vi "Modbus RT Driver VI Modbus - Read Write Items.vi"(5 "DEBUG RT-FIFOs Indexes":T1[](array[typedef]), 7 "DEBUG Modbus Items":T3[](array[typedef]), 8 "error in (no error)":errorcluster, 9 "Inputs In":dbl[](array[numeric]), 10 "Outputs In":dbl[](array[numeric]), 11 "ModbusPharLap.lvlibp:Modbus API":refnum<class "Modbus API.lvclass">) -> (0 "error out":errorcluster, 2 "Outputs Out":dbl[](array[numeric]), 3 "ModbusPharLap.lvlibp:Modbus API":refnum<class "Modbus API.lvclass">)   [LabVIEW 2014, in "Modbus Engine.lvlib"]
uses:
  Modbus Engine.lvlib
  XML Deserializer/XML VIs/API/Controls/Modbus_Items.ctl
  XML Deserializer/XML VIs/API/Controls/Modbus_Item_Type.ctl
  Shared/FIFO Indexes.ctl
  <vilib>/NI Veristand/Custom Device API/Custom Device Channel Type.ctl
  ModbusPharLap.lvlibp/Modbus Library/API/Modbus API.lvclass
  ModbusPharLap.lvlibp/Modbus Library/API/Slave/Modbus Slave.lvclass
  Shared/Modbus Shared.lvlib
  <vilib>/NI Veristand/Custom Device API/Custom Device API.lvlib
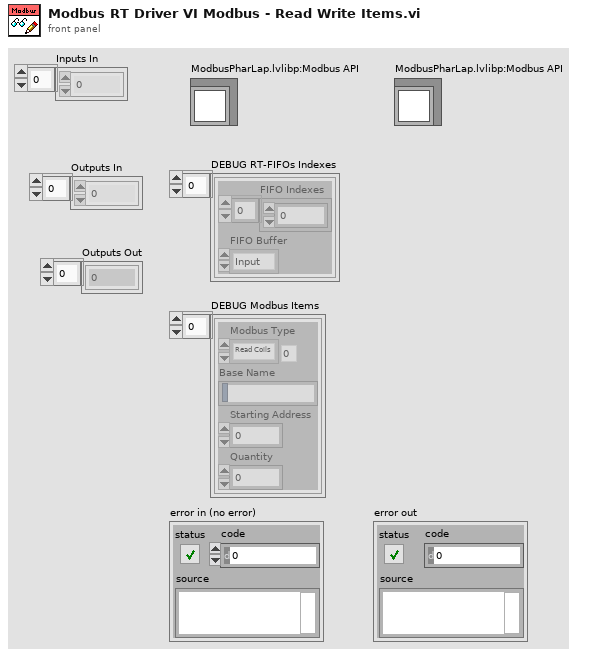
[diagram p1: front panel]
types:
  T1 = typedef "Modbus Shared.lvlib/FIFO Indexes.ctl" = cluster{"FIFO Indexes":i32[], "FIFO Buffer":T2}
  T2 = typedef "Custom Device API.lvlib/Custom Device Channel Type.ctl" = enum16{"Input", "Output"}
  T3 = typedef "Modbus Shared.lvlib/Modbus_Items.ctl" = cluster{"Modbus Type":T4, "Base Name":string, "Starting Address":u16, "Quantity":u16}
  T4 = typedef "Modbus Shared.lvlib/Modbus_Item_Type.ctl" = enum16{"Read Coils", "Read Discrete Inputs", "Read Holding Registers", "Read Input Registers", "Write Multiple Coils", "Write Multiple Holding Registers", "Write Single Coil", "Write Single Holding Register", "Write Multiple Discrete Inputs", "Write Multiple Input Registers"}
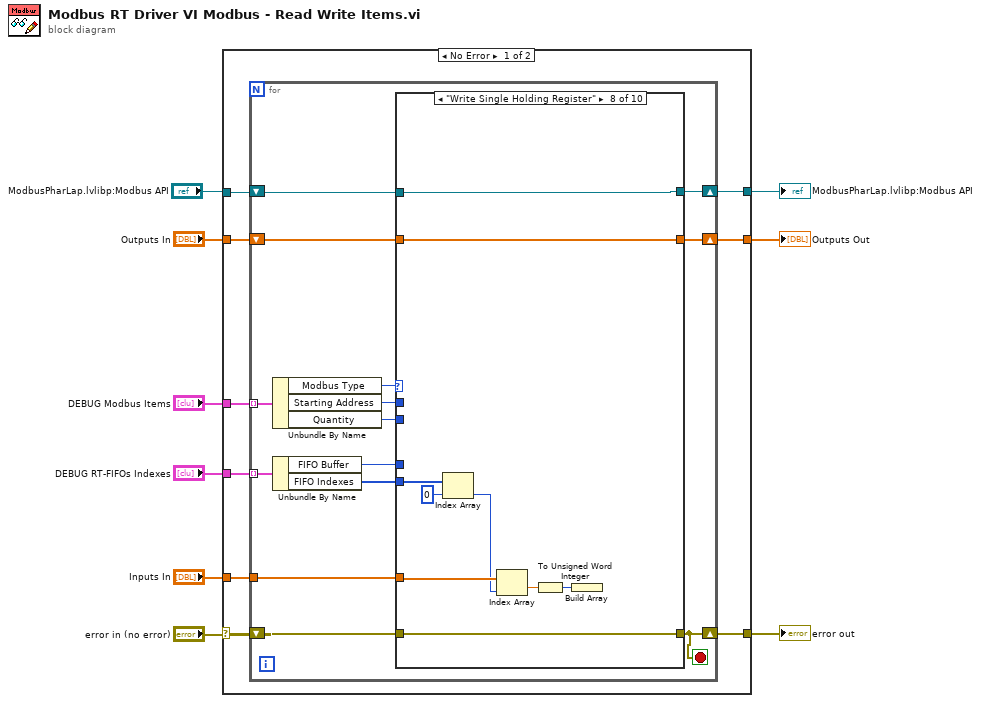
[diagram p0: block diagram]
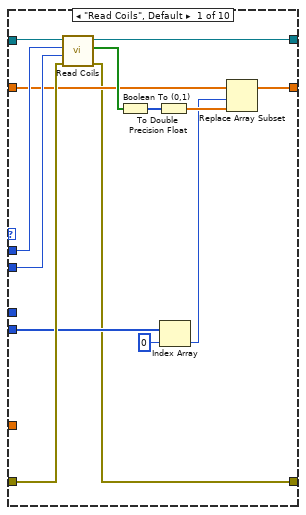
[diagram p2: hidden frame]
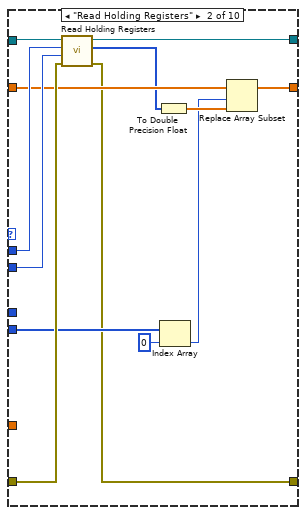
[diagram p3: hidden frame]
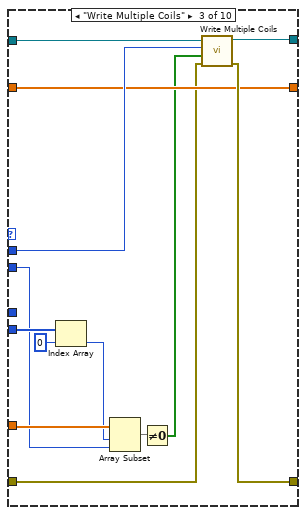
[diagram p4: hidden frame]
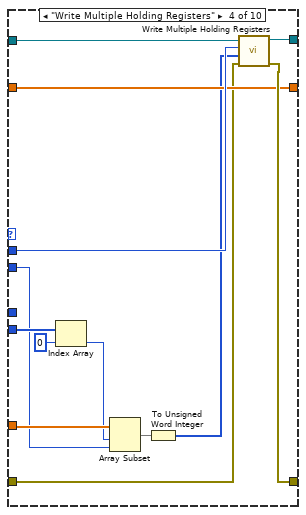
[diagram p5: hidden frame]
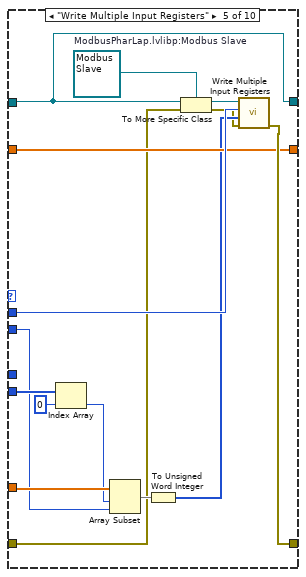
[diagram p6: hidden frame]
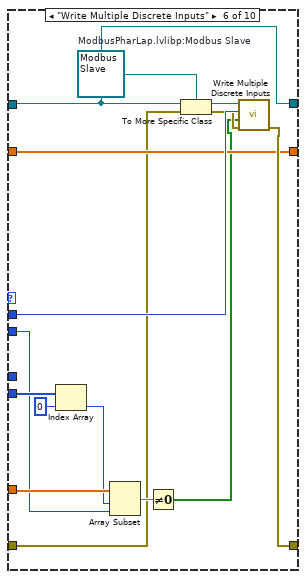
[diagram p7: hidden frame]
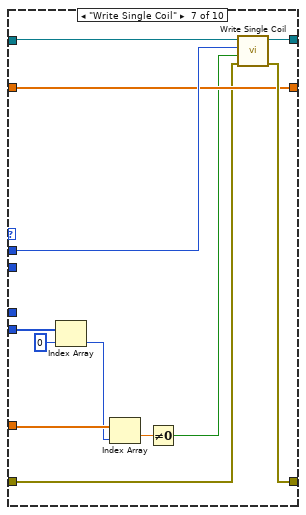
[diagram p8: hidden frame]
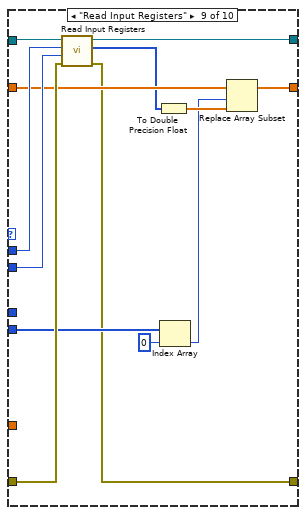
[diagram p9: hidden frame]
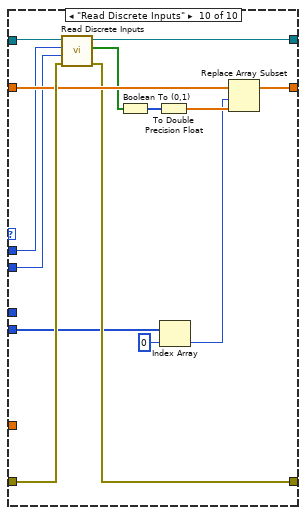
[diagram p10: hidden frame]
diagram:
  n1 = case shown="No Error" "error in (no error)" {
    selector: "error in (no error)" -> [w16 w166]
    tunnel: [w15 w166] -> w8
    tunnel: "ModbusPharLap.lvlibp:Modbus API" -> [w11 w165]
    tunnel: [w10 w165] -> w2
    tunnel: "Outputs In" -> [w14 w164]
    tunnel: [w12 w164] -> w6
    tunnel: "Inputs In" -> [w13 _]
    tunnel: "DEBUG Modbus Items" -> [w18 _]
    tunnel: "DEBUG RT-FIFOs Indexes" -> [w17 _]
    frame No Error {
      n2 = for {
        tunnel: w18 -> [w32] mode=indexing
        tunnel: w17 -> [w31] mode=indexing
        shift-right: [w20] -> w15
        shift-left: w16 -> [w26]
        shift-right: [w21] -> w12
        shift-left: w14 -> [w24]
        tunnel: w13 -> [w25]
        shift-right: [w19] -> w10
        shift-left: w11 -> [w29]
        stop <- w20 stop-if-true
        n3 = Unbundle By Name(w32) -> ("Modbus Type"=w30:T4, "Starting Address"=w28:u16, "Quantity"=w27:u16)
        n4 = Unbundle By Name(w31) -> ("FIFO Buffer"=w23:T2, "FIFO Indexes"=w22:i32[])
        n5 = case shown="\"Write Single Holding Register\"" w30 {
          tunnel: w29 -> [w34 w48 w61 w75 w87 w102 w117 w129 w138 w151]
          tunnel: w28 -> [w46 w59 w72 w85 w100 w115 w127 _ w149 w157]
          tunnel: w27 -> [w45 w58 w65 w78 w93 w108 _ _ w148 w156]
          tunnel: w26 -> [w44 w57 w62 w74 w90 w106 w119 w128 w147 w163]
          tunnel: w25 -> [_ _ w67 w80 w95 w110 w122 w133 _ _]
          tunnel: w24 -> [w41 w56 w68 w81 w96 w111 w123 w134 w146 w162]
          tunnel: w23 -> [_ _ _ _ _ _ _ _ _ _]
          tunnel: w22 -> [w38 w53 w71 w84 w99 w114 w126 w136 w143 w153]
          tunnel: [w40 w55 w68 w81 w96 w111 w123 w134 w145 w161] -> w21
          tunnel: [w35 w50 w69 w82 w97 w112 w124 w128 w140 w158] -> w20
          tunnel: [w33 w47 w60 w73 w87 w102 w116 w129 w137 w150] -> w19
          frame "Read Coils", Default {
            n6 = call-dynamic "Read Coils.vi"("error in"=w44, "number of inputs"=w45, "starting address"=w46, "Modbus instance in"=w34) -> ("error out"=w35:errorcluster, "coils"=w43:bool[], "Modbus instance out"=w33:refnum<class "Modbus API.lvclass">)  [unwired: 5 in]
            n7 = Boolean To (0,1)(Boolean=w43) -> (0, 1=w42:i16[])
            n8 = To Double Precision Float(number=w42) -> (double precision float=w39:dbl[])
            n9 = Index Array(array=w38, index=0) -> (element=w36:i32)
            n10 = Replace Array Subset(array=w41, new element=w39, index=w36) -> (w40:dbl[])
          }
          frame "Read Holding Registers" {
            n11 = call-dynamic "Read Holding Registers.vi"("error in"=w57, "number of inputs"=w58, "starting address"=w59, "Modbus instance in"=w48) -> ("error out"=w50:errorcluster, "register values"=w49:u16[], "Modbus instance out"=w47:refnum<class "Modbus API.lvclass">)  [unwired: 5 in]
            n12 = To Double Precision Float(number=w49) -> (double precision float=w54:dbl[])
            n13 = Index Array(array=w53, index=0) -> (element=w51:i32)
            n14 = Replace Array Subset(array=w56, new element=w54, index=w51) -> (w55:dbl[])
          }
          frame "Write Multiple Coils" {
            n15 = Index Array(array=w71, index=0) -> (element=w66:i32)
            n16 = Array Subset(array=w67, index=w66, length=w65) -> (w64:dbl[])
            n17 = Not Equal To 0?(x=w64) -> (x != 0?=w63:bool[])
            n18 = call-dynamic "Write Multiple Coils.vi"("error in"=w62, "coils to write"=w63, "starting address"=w72, "Modbus instance in"=w61) -> ("error out"=w69:errorcluster, "Modbus instance out"=w60:refnum<class "Modbus API.lvclass">)  [unwired: 6 in]
          }
          frame "Write Multiple Holding Registers" {
            n19 = Index Array(array=w84, index=0) -> (element=w79:i32)
            n20 = Array Subset(array=w80, index=w79, length=w78) -> (w77:dbl[])
            n21 = To Unsigned Word Integer(number=w77) -> (unsigned 16bit integer=w76:u16[])
            n22 = call-dynamic "Write Multiple Holding Registers.vi"("error in"=w74, "registers to write"=w76, "starting address"=w85, "Modbus instance in"=w75) -> ("error out"=w82:errorcluster, "Modbus instance out"=w73:refnum<class "Modbus API.lvclass">)  [unwired: 6 in]
          }
          frame "Write Multiple Input Registers" {
            w86 = refnum<class "Modbus Slave.lvclass"> refnum  # ModbusPharLap.lvlibp:Modbus Slave
            n23 = Index Array(array=w99, index=0) -> (element=w94:i32)
            n24 = Array Subset(array=w95, index=w94, length=w93) -> (w92:dbl[])
            n25 = To Unsigned Word Integer(number=w92) -> (unsigned 16bit integer=w91:u16[])
            n26 = To More Specific Class(target class=w86, reference=w87, error in=w90) -> (specific class reference=w88:refnum<class "Modbus Slave.lvclass">, error out=w89:errorcluster)
            n27 = call-dynamic "Write Multiple Input Registers.vi"("error in"=w89, "input registers to write"=w91, "starting address"=w100, "Modbus slave in"=w88) -> ("error out"=w97:errorcluster)  [unwired: 6 in, 1 out]
          }
          frame "Write Multiple Discrete Inputs" {
            w101 = refnum<class "Modbus Slave.lvclass"> refnum  # ModbusPharLap.lvlibp:Modbus Slave
            n28 = Index Array(array=w114, index=0) -> (element=w109:i32)
            n29 = Array Subset(array=w110, index=w109, length=w108) -> (w107:dbl[])
            n30 = Not Equal To 0?(x=w107) -> (x != 0?=w104:bool[])
            n31 = To More Specific Class(target class=w101, reference=w102, error in=w106) -> (specific class reference=w103:refnum<class "Modbus Slave.lvclass">, error out=w105:errorcluster)
            n32 = call-dynamic "Write Multiple Discrete Inputs.vi"("error in"=w105, "discrete inputs to write"=w104, "starting address"=w115, "Modbus slave in"=w103) -> ("error out"=w112:errorcluster)  [unwired: 6 in, 1 out]
          }
          frame "Write Single Coil" {
            n33 = Index Array(array=w126, index=0) -> (element=w121:i32)
            n34 = Index Array(array=w122, index=w121) -> (element=w120:dbl)
            n35 = Not Equal To 0?(x=w120) -> (x != 0?=w118:bool)
            n36 = call-dynamic "Write Single Coil.vi"("error in"=w119, "coil to write"=w118, "address"=w127, "Modbus instance in"=w117) -> ("error out"=w124:errorcluster, "Modbus instance out"=w116:refnum<class "Modbus API.lvclass">)  [unwired: 6 in]
          }
          frame "Write Single Holding Register" {
            n37 = Index Array(array=w136, index=0) -> (element=w132:i32)
            n38 = Index Array(array=w133, index=w132) -> (element=w131:dbl)
            n39 = To Unsigned Word Integer(number=w131) -> (unsigned 16bit integer=w130:u16)
            n40 = Build Array(w130) -> ()  [unwired: 1 out]
          }
          frame "Read Input Registers" {
            n41 = call-dynamic "Read Input Registers.vi"("error in"=w147, "number of inputs"=w148, "starting address"=w149, "Modbus instance in"=w138) -> ("error out"=w140:errorcluster, "register values"=w139:u16[], "Modbus instance out"=w137:refnum<class "Modbus API.lvclass">)  [unwired: 5 in]
            n42 = To Double Precision Float(number=w139) -> (double precision float=w144:dbl[])
            n43 = Index Array(array=w143, index=0) -> (element=w141:i32)
            n44 = Replace Array Subset(array=w146, new element=w144, index=w141) -> (w145:dbl[])
          }
          frame "Read Discrete Inputs" {
            n45 = call-dynamic "Read Discrete Inputs.vi"("error in"=w163, "number of inputs"=w156, "starting address"=w157, "Modbus instance in"=w151) -> ("error out"=w158:errorcluster, "discrete inputs"=w154:bool[], "Modbus instance out"=w150:refnum<class "Modbus API.lvclass">)  [unwired: 5 in]
            n46 = Boolean To (0,1)(Boolean=w154) -> (0, 1=w155:i16[])
            n47 = To Double Precision Float(number=w155) -> (double precision float=w160:dbl[])
            n48 = Index Array(array=w153, index=0) -> (element=w152:i32)
            n49 = Replace Array Subset(array=w162, new element=w160, index=w152) -> (w161:dbl[])
          }
        }
      }
    }
    frame Error {
    }
  }
  "error out" <- w8
  "Outputs Out" <- w6
  "ModbusPharLap.lvlibp:Modbus API" <- w2
